vi "Gets APU Column Index.vi"(6 "Numeric Vals?":bool, 8 "error in (no error)":errorcluster, 9 "Tag":string, 10 "[Column Names]":string[](array[string]), 11 "[[Array of Info]]":string[][](array[string])) -> (0 "error out":errorcluster, 1 "Row Index":i32, 2 "[Col Indices]":i32[](array[numeric]), 3 "[Values out]":string[](array[string]), 4 "Numeric Vals":dbl[](array[numeric]))   [LabVIEW 2018]
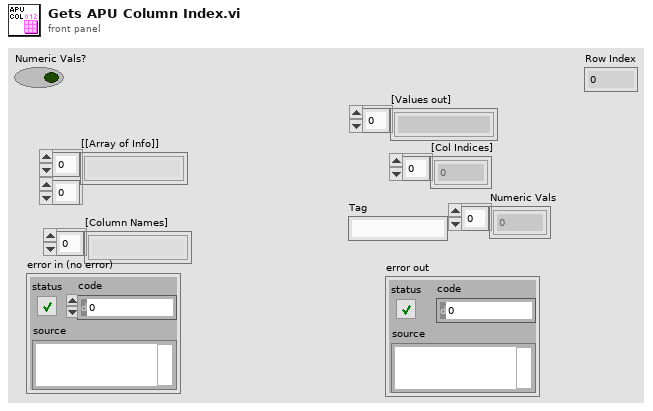
[diagram p1: front panel]
types:
  T1 = cluster{"[[Array of Info]]":string[][], "Tag":string, "[Column Names]":string[]}
  T2 = cluster{"index of element":i32, i32[], string[], dbl[]}
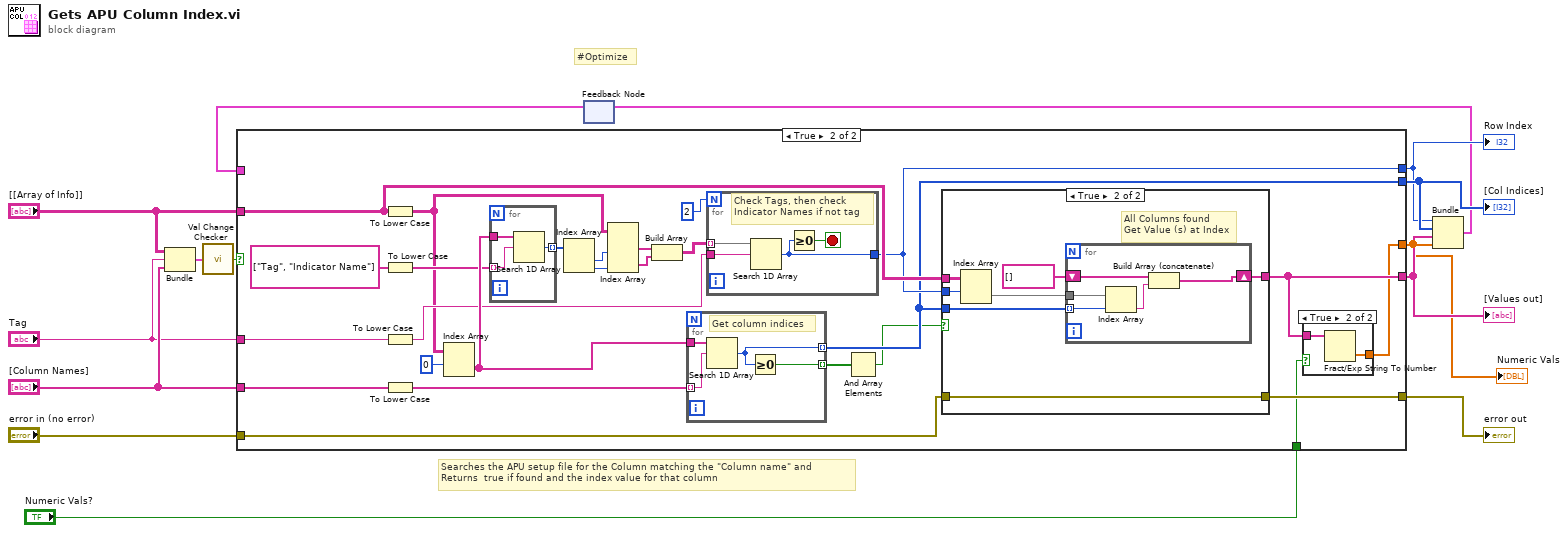
[diagram p0: block diagram]
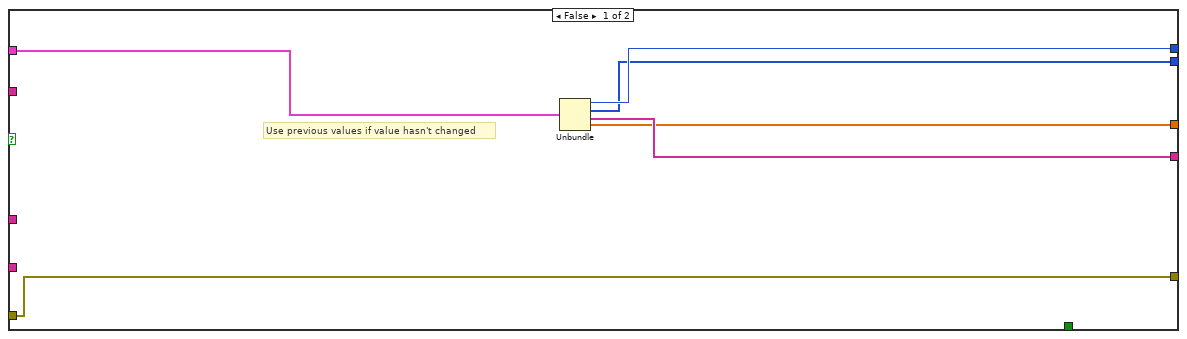
[diagram p2: hidden frame]
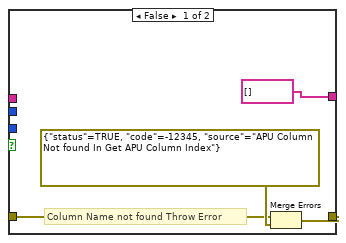
[diagram p4: hidden frame]
diagram:
  # "#Optimize"
  # "Searches the APU setup file for the Column matching the \"Column name\" and\nReturns  true if found and the index value for that column"
  n1 = Bundle("[[Array of Info]]"="[[Array of Info]]", "Tag"="Tag", "[Column Names]"="[Column Names]") -> (w11:T1)  [unwired: 1 in]
  n2 = call "Val Change Checker.vi"("Current Value in"=w11) -> ("Value Change?"=w10:bool)
  n3 = feedback #1() -> (w6:T2)  [unwired: 1 in]
  n4 = case shown="True" w10 {
    tunnel: [w18 w27] -> w9
    tunnel: "Tag" -> [_ w44]
    tunnel: [w19 w28] -> w8
    tunnel: "[Column Names]" -> [_ w35]
    tunnel: "[[Array of Info]]" -> [_ w29]
    tunnel: w6 -> [w20 _]
    tunnel: "error in (no error)" -> [w17 w26]
    tunnel: [w16 w22] -> w3
    tunnel: [w17 w24] -> w4
    tunnel: "Numeric Vals?" -> [_ w23]
    tunnel: [w15 w21] -> w1
    frame False {
      # "Use previous values if value hasn't changed"
      n5 = Unbundle(w20) -> ("index of element"=w19:i32, w18:i32[], w16:string[], w15:dbl[])
    }
    frame True {
      n6 = To Lower Case(string=w29) -> (all lower case string=w30:string[][])
      n7 = To Lower Case(string=string[] ["Tag", "Indicator Name"] ("[Column Names]")) -> (all lower case string=w33:string[])
      n8 = To Lower Case(string=w44) -> (all lower case string=w32:string)
      n9 = To Lower Case(string=w35) -> (all lower case string=w31:string[])
      n10 = Index Array(array=w30, index (row)=0) -> (element=w39:string[])  [unwired: 1 in]
      n11 = for {
        tunnel: w39 -> [w67]
        tunnel: w33 -> [w65] mode=indexing
        tunnel: [w66] -> w38 mode=indexing
        n12 = Search 1D Array(1D array=w67, element=w65) -> (index of element=w66:i32)  [unwired: 1 in]
      }
      n13 = Index Array(array=w38) -> (element #1=w37:i32, element #2=w36:i32)  [unwired: 2 in]
      n14 = Index Array(array=w30, index (col) #1=w37, index (col) #2=w36) -> (element #1=w42:string[], element #2=w40:string[])  [unwired: 2 in]
      n15 = Build Array(w42, w40) -> (w41:string[][])
      n16 = for {
        tunnel: w39 -> [w75]
        tunnel: w31 -> [w72] mode=indexing
        tunnel: [w73] -> w45 mode=indexing
        tunnel: [w74] -> w27 mode=indexing
        # "Get column indices"
        n17 = Search 1D Array(1D array=w75, element=w72) -> (index of element=w74:i32)  [unwired: 1 in]
        n18 = Greater Or Equal To 0?(x=w74) -> (x >= 0?=w73:bool)
      }
      n19 = for {
        N: 2 -> [_]
        tunnel: w32 -> [w71]
        tunnel: [w70] -> w28
        tunnel: w41 -> [w68] mode=indexing
        stop <- w69 stop-if-true
        # "Check Tags, then check\nIndicator Names if not tag"
        n20 = Search 1D Array(1D array=w68, element=w71) -> (index of element=w70:i32)  [unwired: 1 in]
        n21 = Greater Or Equal To 0?(x=w70) -> (x >= 0?=w69:bool)
      }
      n22 = And Array Elements(Boolean array=w45) -> (logical AND=w25:bool)
      n23 = case shown="True" w25 {
        tunnel: w26 -> [w49 w59]
        tunnel: [w50 w59] -> w24
        tunnel: w28 -> [_ w57]
        tunnel: w29 -> [_ w58]
        tunnel: w27 -> [_ w56]
        tunnel: [string[] [] w53] -> w22
        frame False {
          # "Column Name not found Throw Error"
          n24 = Merge Errors(w49, errorcluster {"status"=TRUE, "code"=-12345, "source"="APU Column Not found In Get APU Column Index"} ("error in (no error)")) -> (w50:errorcluster)
        }
        frame True {
          # "All Columns found\nGet Value (s) at Index"
          n25 = Index Array(array=w58, index (row)=w57) -> (element=w55:string[])  [unwired: 1 in]
          n26 = for {
            tunnel: w56 -> [w63] mode=indexing
            tunnel: w55 -> [w64]
            shift-right: [w61] -> w53
            shift-left: string[] [] -> [w60]
            n27 = Index Array(array=w64, index=w63) -> (element=w62:string)
            n28 = Build Array (concatenate)(w60, w62) -> (w61:string[])
          }
        }
      }
      n29 = case shown="True" w23 {
        tunnel: w22 -> [_ w48]
        tunnel: [_ w47] -> w21
        frame False {
        }
        frame True {
          n30 = Fract/Exp String To Number(string=w48) -> (number=w47:dbl[])  [unwired: 3 in, 1 out]
        }
      }
    }
  }
  "error out" <- w4
  "[Values out]" <- w3
  "[Col Indices]" <- w9
  "Row Index" <- w8
  "Numeric Vals" <- w1
  n31 = Bundle("index of element"=w8, w9, w3, w1) -> (w7:T2)  [unwired: 1 in]
  n32 = feedback-in #1(w7) -> ()
